vi "HK Channel Initialize.vi"(8 "error in (no error)":errorcluster, 9 "Channel Configuration File":path, 10 "CVT Settings":T1 {"Max Age" format="%<%H:%M:%S>t"}, 11 "HK Channel in":refnum<class "HK Table.lvclass">) -> (0 "error out":errorcluster, 3 "HK Channel out":refnum<class "HK Table.lvclass">)   [LabVIEW 2024, in "HK Table.lvclass"]
uses:
  HK Table.lvclass
  HK Current Value Table Settings.ctl
  HK Item/HK Item.lvclass
  HK Current Value Table Element.ctl
  HK Alarms/HK Alarm enum Status.ctl
  HK Table.lvclass/HK Table.ctl
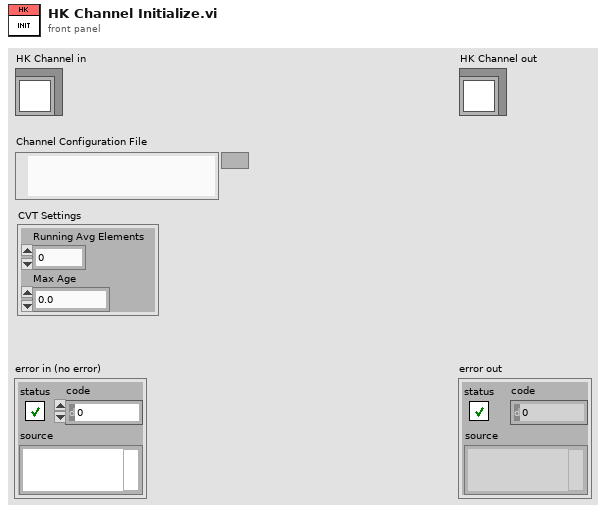
[diagram p1: front panel]
types:
  T1 = typedef "HK Table.lvclass/HK Current Value Table Settings.ctl" = cluster{"Running Avg Elements":i32, "Max Age":dbl}
  T2 = typedef "HK Table.lvclass/HK Current Value Table Element.ctl" = cluster{"Value":dbl, "Time Stamp":timestamp, "Running Avg.":dbl, "Std. Dev.":dbl, "Recent Values":dbl[], "Timestamps":timestamp[], "Alarm Status":T3}
  T3 = typedef "HK Item.lvclass/HK Alarm enum Status.ctl" = enum16{"No Alarm", "Red Low", "Red High", "Yellow Low", "Yellow High"}
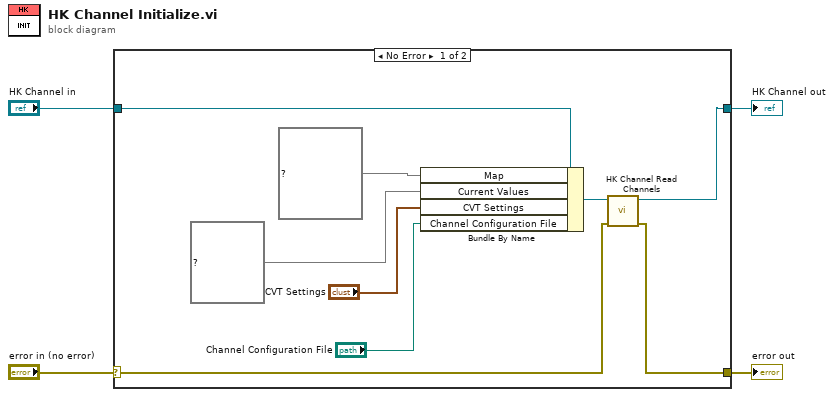
[diagram p0: block diagram]
diagram:
  n1 = case shown="No Error" "error in (no error)" {
    selector: "error in (no error)" -> [w6 w15]
    tunnel: [w5 w15] -> w3
    tunnel: [w7 w14] -> w1
    tunnel: "HK Channel in" -> [w13 w14]
    frame No Error {
      n2 = Bundle By Name(cluster=w13, "Map"=map{string, refnum<class "HK Item.lvclass">} {}, "Current Values"=map{string, T2} {}, "CVT Settings"="CVT Settings", "Channel Configuration File"="Channel Configuration File") -> (w8:refnum<class "HK Table.lvclass">)
      n3 = call-dynamic "HK Channel Read Channels.vi"("error in (no error)"=w6, "HK Channel in"=w8) -> ("error out"=w5:errorcluster, "HK Channel out"=w7:refnum<class "HK Table.lvclass">)  [unwired: 8 in]
    }
    frame Error {
    }
  }
  "error out" <- w3
  "HK Channel out" <- w1
